vi "Temp Sweep Control.vi"() -> ()   [LabVIEW 2016, in "Transport.lvclass"]
uses:
  Transport.lvclass
  Control Experiment SM/Control Experiment SM.lvclass
  <userlib>/LevyLab/Levylab Instruments/Instrument Types/Cryostat/Instrument.Cryostat.lvclass
panel:
  out "Current State":string
  in  "Wait time":dbl
  in  "T Start (K)":i32=275
  in  "T Step (K)":i32=5
  in  "Number":i32=26
  out "sequence":string
  in  "simulate?":bool
  in  "Start":bool
  in  "OK":bool
  in  "Experiment Description":string
  in  "Experiment Folder (## - Description)":string="00 - test"
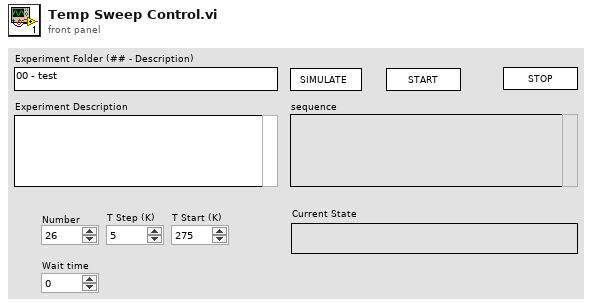
[diagram p1: front panel]
types:
  T1 = enum32{"Invalid", "Standard", "Closed", "Hidden", "Minimized", "Maximized"}
  T2 = enum32{"invalid app kind", "Development System", "Run Time System", "Student Edition", "Embedded LabVIEW", "Evaluation", "Custom"}
  T3 = cluster{"Core":cluster{"Current VI Reference":refnum<vi>, "Close Panel on Exit?":bool}, "C.E.":refnum<class "Control Experiment SM.lvclass">, "notifier":refnum<notifier>, "Lockin Start":timestamp, "Temp":dbl, "Wait time":dbl}
  T4 = cluster{"Current VI Reference":refnum<vi>, "Close Panel on Exit?":bool}
  T5 = typedef "Control Experiment SM.lvclass/Instruments--cluster.ctl" = cluster{"KH7008":refnum<class "Instrument.KH7008.lvclass">[], "Lockin":refnum<class "Instrument.Lockin.lvclass">, "Temperature":refnum<class "Instrument.Cryostat.lvclass">, "Magnet":refnum<class "Instrument.Cryostat.lvclass">, "Rotator":refnum<class "Instrument.Cryostat.lvclass">, "Level":refnum<class "Instrument.Cryostat.lvclass">, "Capacitance Bridge":refnum<class "Instrument.CBridge.lvclass">, "Optical Delay Line":refnum<class "Instrument.OpticalDelayLine.lvclass">, "Strain Cell":refnum<class "Instrument.Strain.lvclass">, "VNA":refnum<class "Instrument.VNA.lvclass">, "Voltage Source":refnum<class "Instrument.VSource.lvclass">}
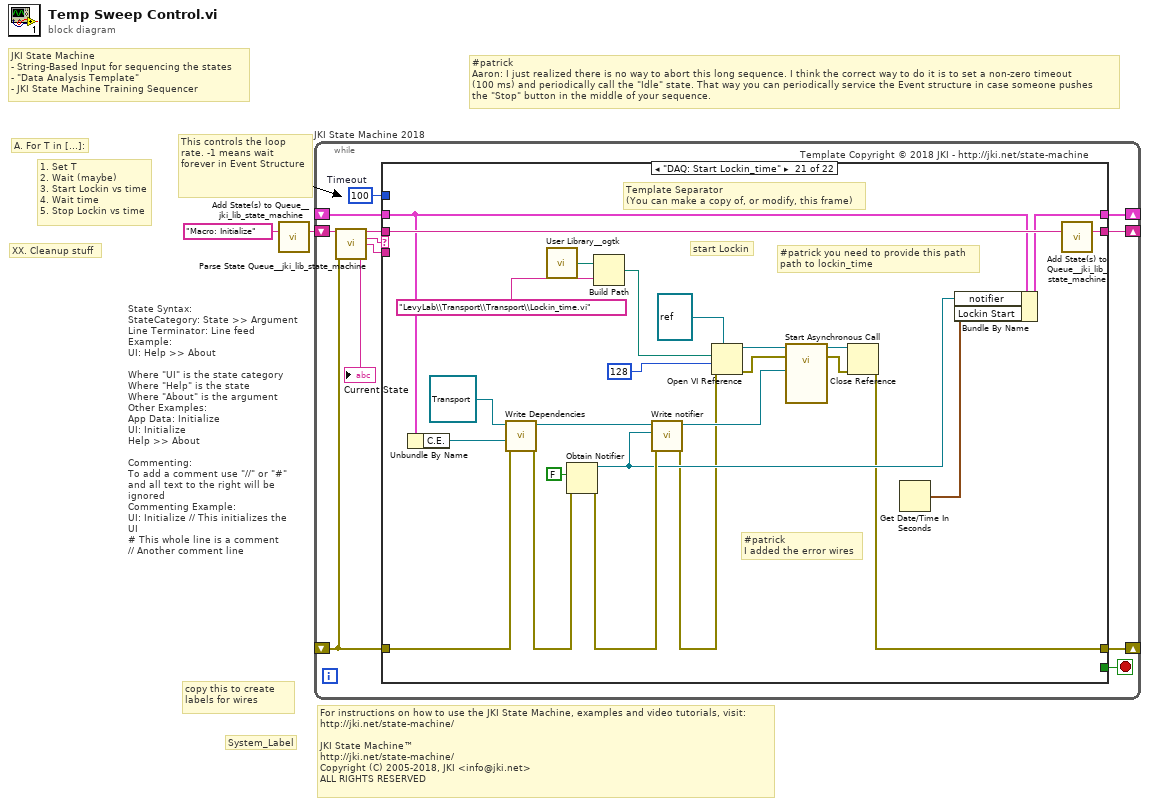
[diagram p0: block diagram]
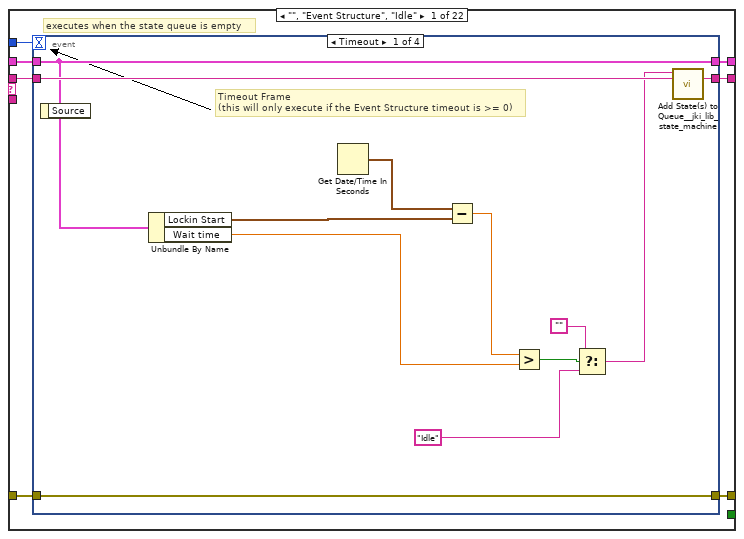
[diagram p2: hidden frame]
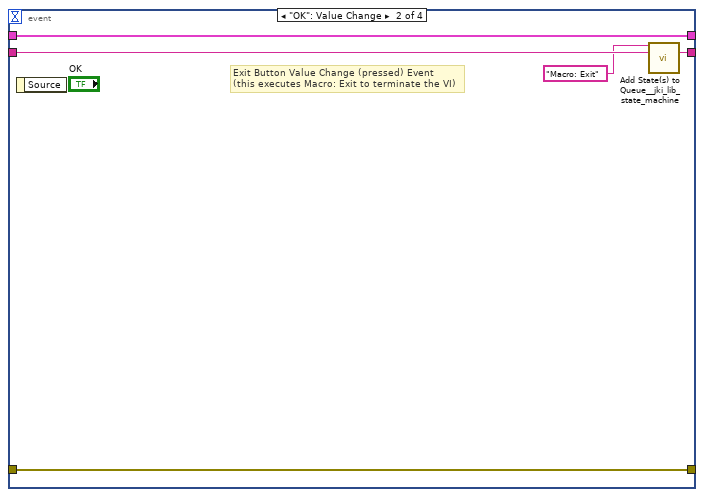
[diagram p3: hidden frame]
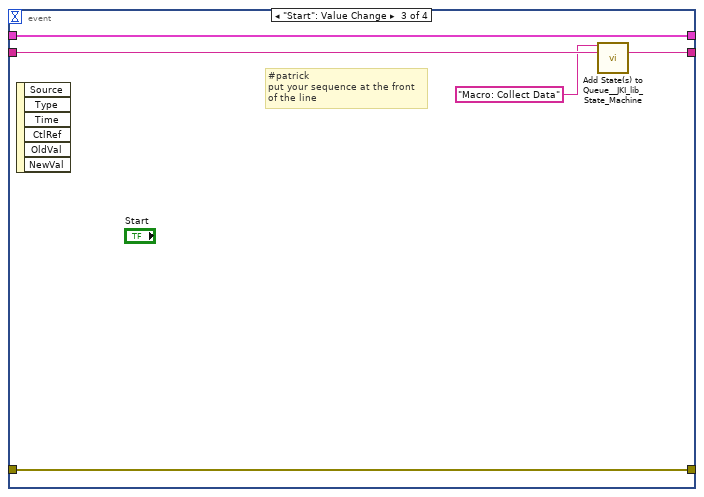
[diagram p4: hidden frame]
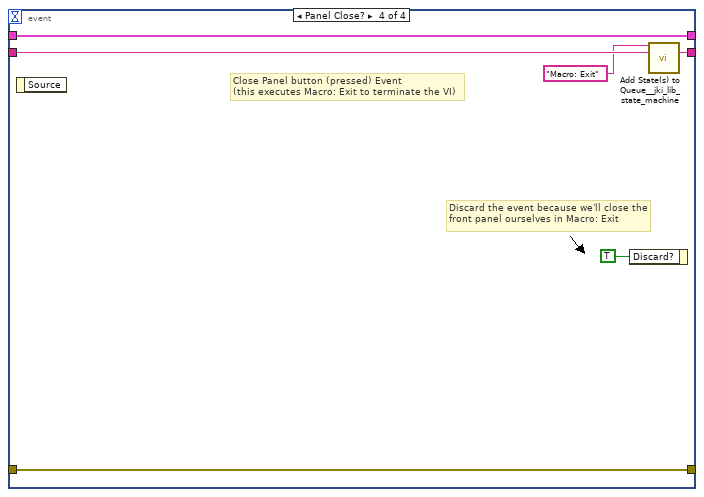
[diagram p5: hidden frame]
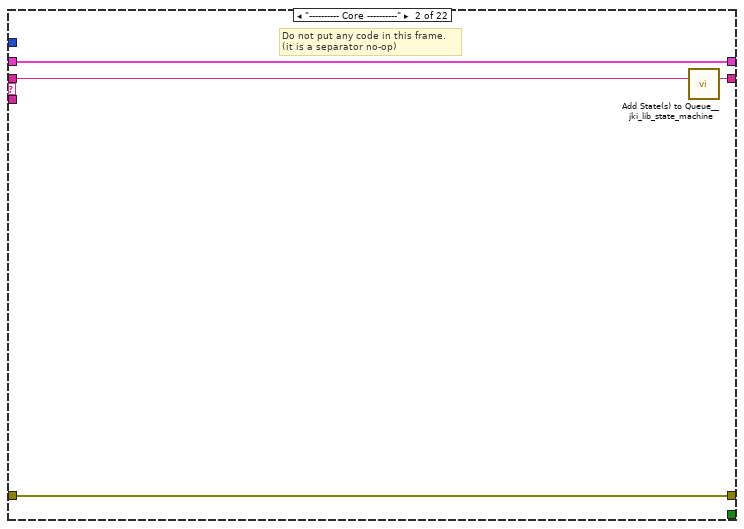
[diagram p6: hidden frame]
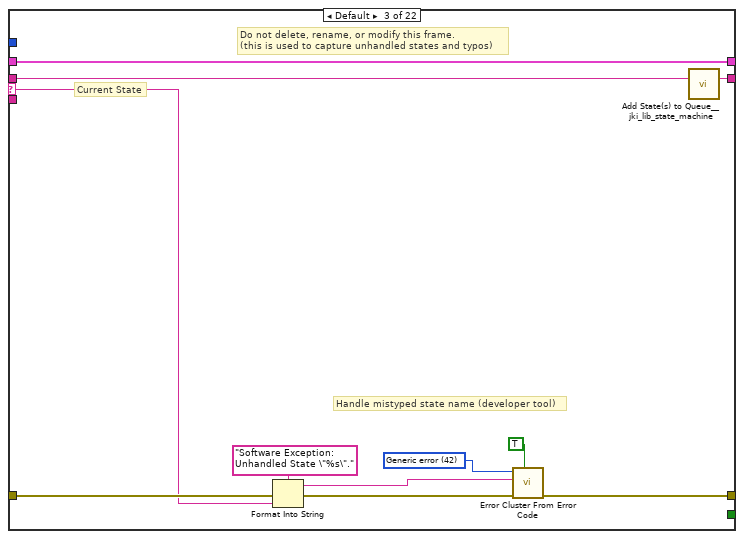
[diagram p7: hidden frame]
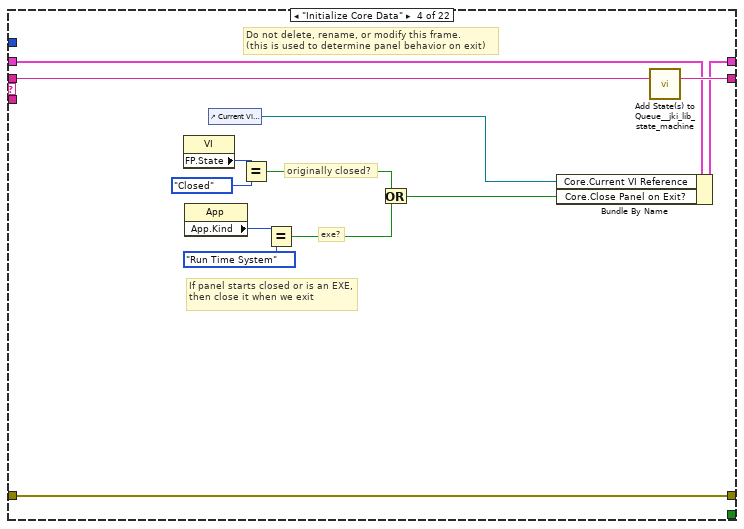
[diagram p8: hidden frame]
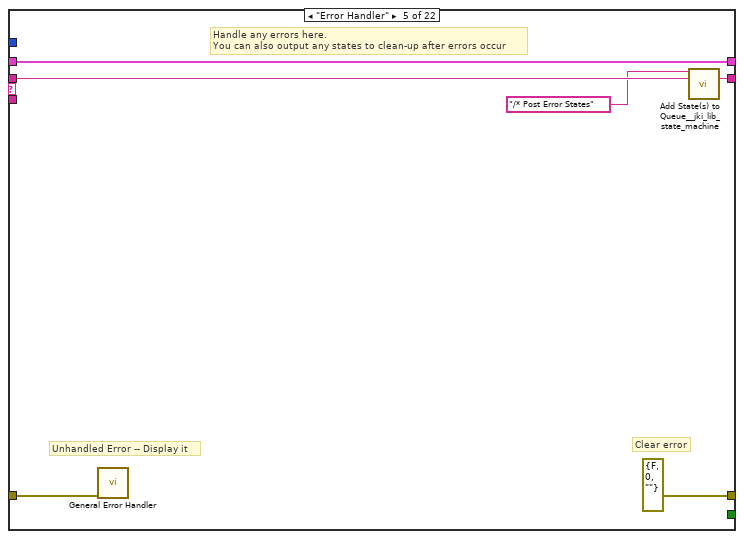
[diagram p9: hidden frame]
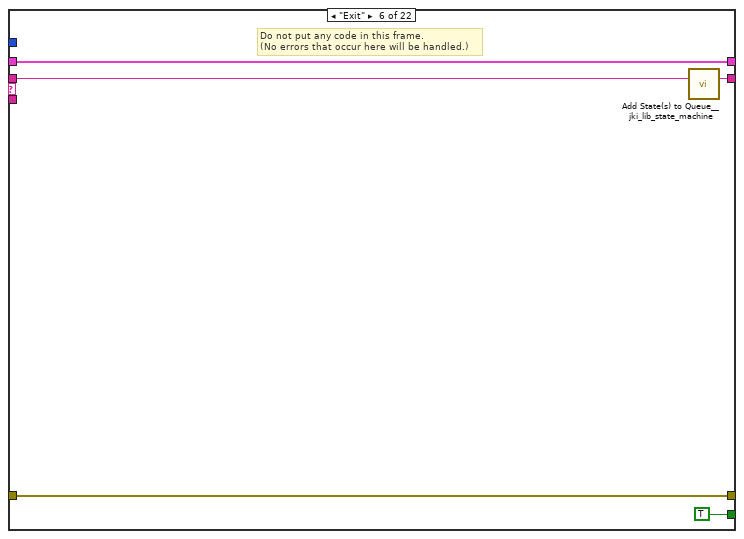
[diagram p10: hidden frame]
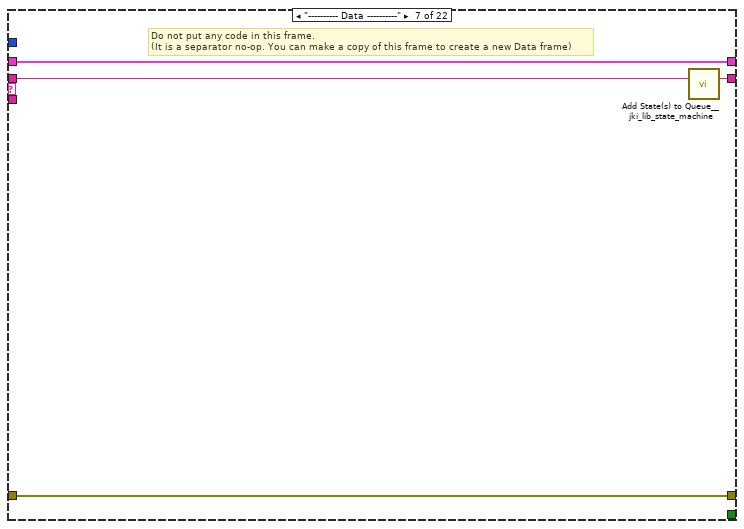
[diagram p11: hidden frame]
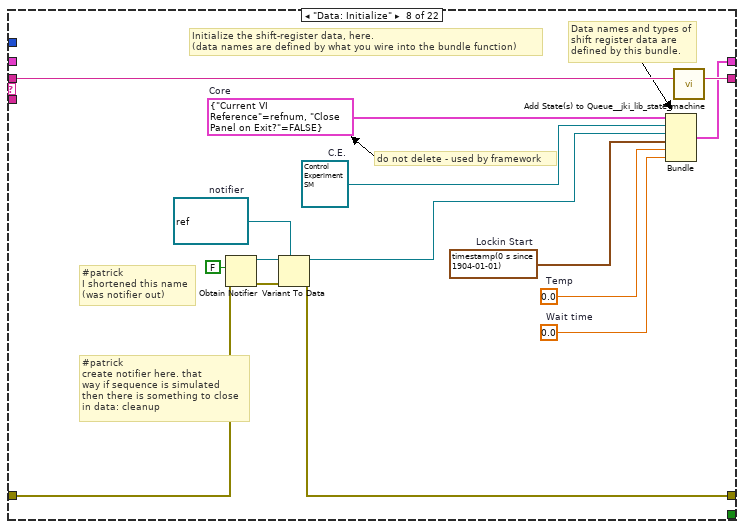
[diagram p12: hidden frame]
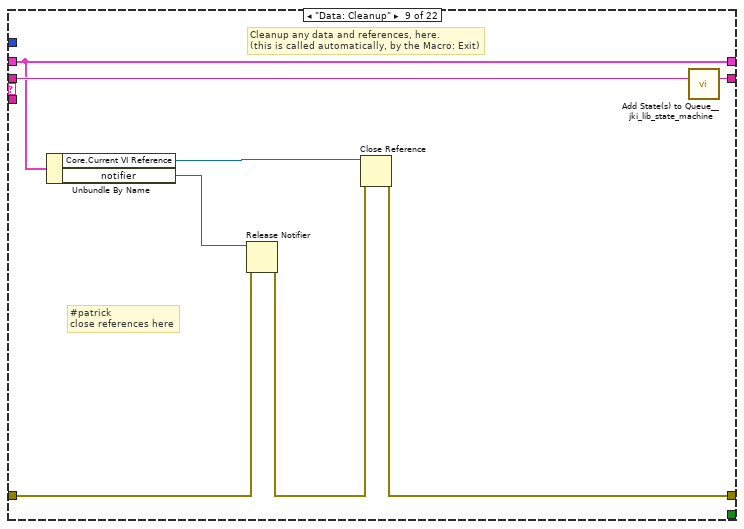
[diagram p13: hidden frame]
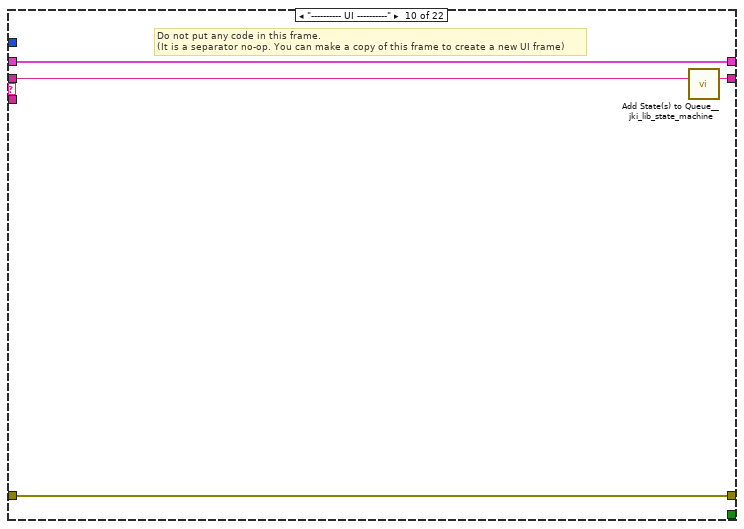
[diagram p14: hidden frame]
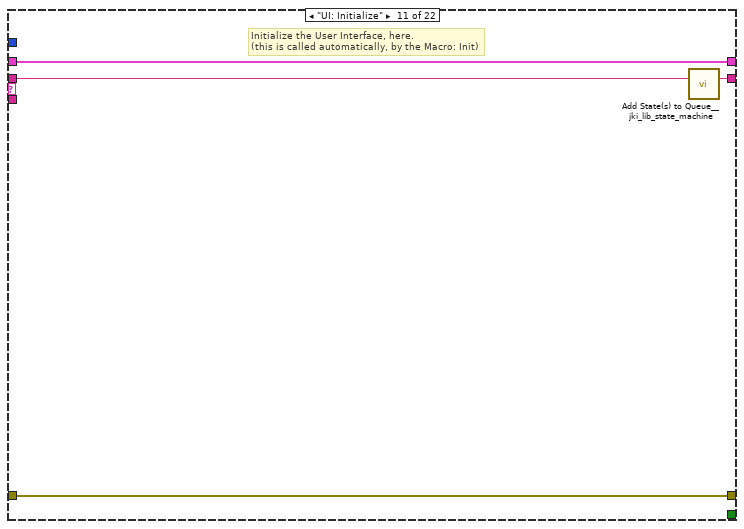
[diagram p15: hidden frame]
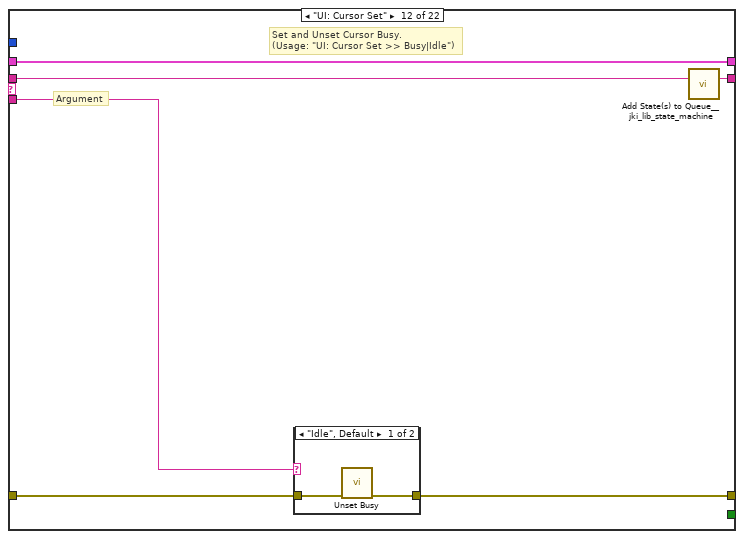
[diagram p16: hidden frame]
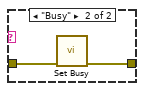
[diagram p17: hidden frame]
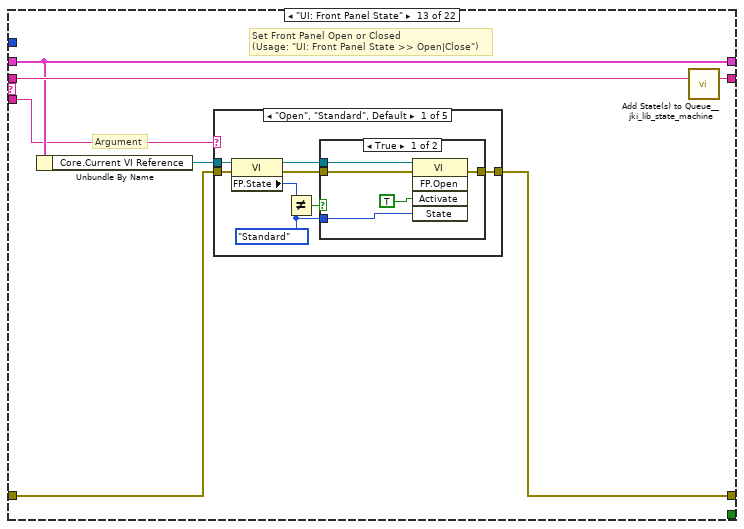
[diagram p18: hidden frame]
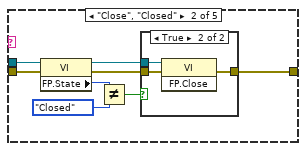
[diagram p20: hidden frame]
diagram:
  # "#patrick\nAaron: I just realized there is no way to abort this long sequence. I think the correct way to do it is to set a non-zero timeout\n(100 ms) and periodically call the \"Idle\" state. That way you can periodically service the Event structure in case someone pushes\nthe \"Stop\" button in the middle of your sequence."
  # "For instructions on how to use the JKI State Machine, examples and video tutorials, visit:\nhttp://jki.net/state-machine/\n\nJKI State Machine™\nhttp://jki.net/state-machine/\nCopyright (C) 2005-2018, JKI <info@jki.net>\nALL RIGHTS RESERVED"
  # "State Syntax:\nStateCategory: State >> Argument\nLine Terminator: Line feed\nExample:\nUI: Help >> About\n\nWhere \"UI\" is the state category\nWhere \"Help\" is the state\nWhere \"About\" is the argument\nOther Examples:\nApp Data: Initialize\nUI: Initialize\nHelp >> About\n\nCommenting:\nTo add a comment use \"//\" or \"#\" and all text to the right will be ignored\nCommenting Example:\nUI: Initialize // This initializes the UI\n# This whole line is a comment\n// Another comment line"
  # "copy this to create labels for wires"
  # "This controls the loop rate. -1 means wait forever in Event Structure"
  # "System_Label"
  # "JKI State Machine\n- String-Based Input for sequencing the states\n- \"Data Analysis Template\"\n- JKI State Machine Training Sequencer"
  # "XX. Cleanup stuff"
  # "A. For T in [...]:"
  # "1. Set T\n2. Wait (maybe)\n3. Start Lockin vs time\n4. Wait time\n5. Stop Lockin vs time"
  n1 = call <vilib>:"Add State(s) to Queue__jki_lib_state_machine.vi"("State(s) in (\"\")"="Macro: Initialize") -> ("States Out"=w2:string)  [unwired: 14 in]
  n2 = while "JKI State Machine 2018" {
    shift-right: [w6] -> _
    shift-left: _ -> [w5]
    shift-right: [w9] -> _
    shift-left: _ -> [w3]
    shift-right: [w8] -> _
    shift-left: w2 -> [w10]
    stop <- w7 stop-if-true
    w4 = 100  # Timeout
    # "Template Copyright © 2018 JKI - http://jki.net/state-machine"
    n3 = call <vilib>:"Parse State Queue__jki_lib_state_machine.vi"("State Queue"=w10, "Error In (no error)"=w3) -> ("Remaining States"=w12:string, "Current State"=w13:string, "Arguments"=w11:string)  [unwired: 11 in]
    "Current State" <- w13
    n4 = case shown="\"DAQ: Start Lockin_time\"" w13 {
      selector: w13 -> [_ _ w53 _ _ _ _ _ _ _ _ _ _ _ _ _ _ _ _ _ _ _]
      tunnel: w12 -> [w20 w52 w57 w76 w82 w87 w91 w106 w114 w118 w122 w128 w139 w208 w213 w226 w248 w252 w267 w284 w320 w327]
      tunnel: w11 -> [_ _ _ _ _ _ _ _ _ _ _ w123 w133 _ _ _ _ _ _ w279 _ _]
      tunnel: w5 -> [w18 w49 w55 w69 w79 w85 w88 _ w110 w115 w120 w126 w135 w205 w210 w223 w245 w249 w254 w278 w310 w325]
      tunnel: [w17 w50 w59 w73 errorcluster {"status"=FALSE, "code"=0, "source"=""} ("error out") w84 w89 w93 w111 w116 w119 w124 w136 w206 w211 w224 w246 w250 w258 w268 w300 w321] -> w9
      tunnel: w3 -> [w16 w50 w58 w73 w78 w84 w89 w94 w108 w116 w119 w125 w137 w206 w211 w224 w246 w250 w256 w276 w306 w322]
      tunnel: [w19 w51 w56 w75 w81 w86 w90 w105 w113 w117 w121 w127 w138 w207 w212 w225 w247 w251 w266 w283 w319 w326] -> w8
      tunnel: [_ _ _ _ _ TRUE _ _ _ _ _ _ _ _ _ _ _ _ _ _ _ _] -> w7
      tunnel: [w15 w49 w55 w74 w79 w85 w88 w104 w110 w115 w120 w126 w135 w205 w210 w223 w245 w249 w255 w277 w312 w325] -> w6
      tunnel: w4 -> [w14 _ _ _ _ _ _ _ _ _ _ _ _ _ _ _ _ _ _ _ _ _]
      frame "", "Event Structure", "Idle" {
        # "executes when the state queue is empty"
        n5 = event shown="[0] Timeout" {
          selector: _ -> [_ _ _ _]
          dyn-events: _ -> [_ _ _ _]
          timeout: w14 -> [_ _ _ _]
          tunnel: w20 -> [w32 w37 w40 w48]
          tunnel: [w31 w36 w39 w47] -> w19
          tunnel: w18 -> [w24 w34 w41 w45]
          tunnel: [w30 w35 w42 w46] -> w17
          tunnel: w16 -> [w30 w35 w42 w46]
          tunnel: [w24 w34 w41 w45] -> w15
          event Timeout {
            # "Timeout Frame\n(this will only execute if the Event Structure timeout is >= 0)"
            n6 = event-data() -> ()  [unwired: 1 in, 1 out]
            n7 = Unbundle By Name(w24) -> ("Lockin Start"=w22:timestamp, "Wait time"=w23:dbl)
            n8 = Get Date/Time In Seconds() -> (seconds since 1Jan1904=w29:timestamp)
            n9 = Subtract(x=w29, y=w22) -> (x-y=w28:dbl)
            n10 = Greater?(x=w28, y=w23) -> (0:w27:bool)
            n11 = Select(t="", s=w27, f="Idle") -> (s? t:f=w21:string)
            n12 = call <vilib>:"Add State(s) to Queue__jki_lib_state_machine.vi"("State(s) in Front (\"\")"=w21, "State(s) in (\"\")"=w32) -> ("States Out"=w31:string)  [unwired: 13 in]
          }
          event "OK": Value Change {
            # "Exit Button Value Change (pressed) Event\n(this executes Macro: Exit to terminate the VI)"
            n13 = event-data() -> ()  [unwired: 1 in, 1 out]
            n14 = call <vilib>:"Add State(s) to Queue__jki_lib_state_machine.vi"("State(s) in Front (\"\")"="Macro: Exit", "State(s) in (\"\")"=w37) -> ("States Out"=w36:string)  [unwired: 13 in]
          }
          event "Start": Value Change {
            # "#patrick\nput your sequence at the front\nof the line"
            n15 = event-data() -> ()  [unwired: 1 in, 6 out]
            n16 = call <vilib>:"Add State(s) to Queue__JKI_lib_State_Machine.vi"("State(s) in Front (\"\")"="Macro: Collect Data", "State(s) in (\"\")"=w40) -> ("States Out"=w39:string)  [unwired: 13 in]
          }
          event Panel Close? {
            # "Discard the event because we'll close the front panel ourselves in Macro: Exit"
            # "Close Panel button (pressed) Event\n(this executes Macro: Exit to terminate the VI)"
            n17 = event-data() -> ()  [unwired: 1 in, 1 out]
            n18 = event-data("Discard?"=TRUE) -> ()  [unwired: 1 in, 1 out]
            n19 = call <vilib>:"Add State(s) to Queue__jki_lib_state_machine.vi"("State(s) in Front (\"\")"="Macro: Exit", "State(s) in (\"\")"=w48) -> ("States Out"=w47:string)  [unwired: 13 in]
          }
        }
      }
      frame "---------- Core ----------" {
        # "Do not put any code in this frame.\n(it is a separator no-op)"
        n20 = call <vilib>:"Add State(s) to Queue__jki_lib_state_machine.vi"("State(s) in (\"\")"=w52) -> ("States Out"=w51:string)  [unwired: 14 in]
      }
      frame Default {
        w62 = 42 items=["No error", "Argument error", "Memory is full", "Out of zone", "End of file", "File already open", "Generic file I/O error", "File not found", "File permission error", "Disk is full", "Duplicate path", "Too many files open", "System feature not enabled", "Resource file not found", "Cannot add resource", "Resource not found", "Image not found", "Image memory error", "Pen does not exist", "Config type invalid", "Config token not found", "Config parse error", "Config memory error", "Bad external code format", "Bad external code offset", "External code not present", "Null window", "Destroy window error", "Null menu", "Print aborted", "Bad print record", "Print driver error", "Windows error during printing", "Memory error during printing", "Print dialog error", "Generic print error", "Invalid device refnum", "Device not found", "Device parameter error", "Device unit error", "Cannot open device", "Device call aborted", "Generic error", "Cancelled by user", "Object ID too low", "Object ID too high", "Object not in heap", "Unknown heap", "Unknown object (invalid DefProc)", "Unknown object (DefProc not in table)", "Message out of range", "Invalid (null) method", "Unknown message", "Manager call not supported", "Bad address", "Network operation in progress", "Network operation timed out", "Connection is busy", "Network attribute not supported", "Network error", "Address in use", "System out of memory", "Connection aborted", "Connection refused", "Not connected", "Already connected", "Connection closed", "Initialization error (interapplication manager)", "Bad occurrence", "Wait on unbound occurrence handler", "Occurrence queue overflow", "Datalog type conflict", "Unused", "Unrecognized type (interapplication manager)", "Memory corrupt", "Failed to make temporary DLL", "Old CIN version", "Drag socket not found", "Failed to load drop-object", "Failed to register OLE object", "Failed to release OLE object", "Format specifier type mismatch", "Unknown format specifier", "Too few format specifiers", "Too many format specifiers", "Scan failed", "Newer CIN version", "Error converting to variant", "Runtime menu error", "Password tampered", "Variant attribute not found", "Incompatible variant data type", "Event data is not available", "Event Store is not present", "Occurrence is not found", "Event Queue is not created", "Event info is not available", "Refnum passed is NULL", "Error retrieving Class GUID", "Error retrieving CoClass GUID", "Error retrieving TypeLib GUID.", "Bad built application magic bytes.", "Specific driver is different from the specific driver associated with the Logical Name.", "There is no session opened to the class driver.", "Max Error", "MAX - Error with config objects", "MAX - Error loading configuration", "MAX - Group not supported"]
        # "Current State"
        # "Do not delete, rename, or modify this frame.\n(this is used to capture unhandled states and typos)"
        # "Handle mistyped state name (developer tool)"
        n21 = Format Into String(format string="Software Exception: Unhandled State \"%s\"." ("message"), error in=w58, w53) -> (resulting string=w61:string, error out=w60:errorcluster)  [unwired: 1 in]
        n22 = call <vilib>:"Error Cluster From Error Code.vi"("show call chain? (False)"=TRUE, "error in (no error)"=w60, "error message (\"\")"=w61, "error code (0)"=w62) -> ("error out"=w59:errorcluster)  [unwired: 5 in]
        n23 = call <vilib>:"Add State(s) to Queue__jki_lib_state_machine.vi"("State(s) in (\"\")"=w57) -> ("States Out"=w56:string)  [unwired: 14 in]
      }
      frame "Initialize Core Data" {
        # "Do not delete, rename, or modify this frame.\n(this is used to determine panel behavior on exit)"
        # "originally closed?"
        # "exe?"
        # "If panel starts closed or is an EXE, then close it when we exit"
        n24 = property class="VI"() -> ("FP.State"=w66:T1)  [unwired: 2 in, 2 out]
        n25 = property class="App"() -> ("App.Kind"=w72:T2)  [unwired: 2 in, 2 out]
        n26 = control-ref of="Current VI Reference"() -> (w67:refnum<vi>)
        n27 = Equal?(x=w66, y=T1."Closed" ("Front Panel Window:State")) -> (x = y?=w64:bool)
        n28 = Equal?(x=w72, y=T2."Run Time System" ("Application:Kind")) -> (x = y?=w70:bool)
        n29 = Or(x=w64, y=w70) -> (x .or. y?=w68:bool)
        n30 = Bundle By Name(cluster=w69, "Core.Current VI Reference"=w67, "Core.Close Panel on Exit?"=w68) -> (w74:T3)
        n31 = call <vilib>:"Add State(s) to Queue__jki_lib_state_machine.vi"("State(s) in (\"\")"=w76) -> ("States Out"=w75:string)  [unwired: 14 in]
      }
      frame "Error Handler" {
        # "Unhandled Error -- Display it"
        # "Handle any errors here.\nYou can also output any states to clean-up after errors occur"
        # "Clear error"
        n32 = call <vilib>:"General Error Handler.vi"("error in (no error)"=w78) -> ()  [unwired: 10 in, 5 out]
        n33 = call <vilib>:"Add State(s) to Queue__jki_lib_state_machine.vi"("State(s) in Front (\"\")"="/* Post Error States", "State(s) in (\"\")"=w82) -> ("States Out"=w81:string)  [unwired: 13 in]
      }
      frame "Exit" {
        # "Do not put any code in this frame.\n(No errors that occur here will be handled.)"
        n34 = call <vilib>:"Add State(s) to Queue__jki_lib_state_machine.vi"("State(s) in (\"\")"=w87) -> ("States Out"=w86:string)  [unwired: 14 in]
      }
      frame "---------- Data ----------" {
        # "Do not put any code in this frame.\n(It is a separator no-op. You can make a copy of this frame to create a new Data frame)"
        n35 = call <vilib>:"Add State(s) to Queue__jki_lib_state_machine.vi"("State(s) in (\"\")"=w91) -> ("States Out"=w90:string)  [unwired: 14 in]
      }
      frame "Data: Initialize" {
        w92 = 0.0  # Wait time
        w100 = 0.0  # Temp
        w101 = timestamp(0 s since 1904-01-01)  # Lockin Start
        w96 = refnum<notifier> refnum  # notifier
        w102 = refnum<class "Control Experiment SM.lvclass"> refnum  # C.E.
        w103 = T4 {"Current VI Reference"=refnum, "Close Panel on Exit?"=FALSE}  # Core
        # "#patrick\ncreate notifier here. that\nway if sequence is simulated\nthen there is something to close\nin data: cleanup"
        # "#patrick\nI shortened this name\n(was notifier out)"
        # "do not delete - used by framework"
        # "Data names and types of shift register data are defined by this bundle."
        # "Initialize the shift-register data, here.\n(data names are defined by what you wire into the bundle function)"
        n36 = Obtain Notifier(notification data type=FALSE, error in (no error)=w94) -> (notifier out=w97:refnum<notifier>, error out=w98:errorcluster)  [unwired: 2 in, 1 out]
        n37 = Variant To Data(error in=w98, type=w96, Variant=w97) -> (data=w95:refnum<notifier>, error out=w93:errorcluster)
        n38 = Bundle("Core"=w103, "C.E."=w102, "notifier"=w95, "Lockin Start"=w101, "Temp"=w100, "Wait time"=w92) -> (w104:T3)  [unwired: 1 in]
        n39 = call <vilib>:"Add State(s) to Queue__jki_lib_state_machine.vi"("State(s) in (\"\")"=w106) -> ("States Out"=w105:string)  [unwired: 14 in]
      }
      frame "Data: Cleanup" {
        # "#patrick\nclose references here"
        # "Cleanup any data and references, here.\n(this is called automatically, by the Macro: Exit)"
        n40 = Unbundle By Name(w110) -> ("Core.Current VI Reference"=w112:refnum<vi>, "notifier"=w109:refnum<notifier>)
        n41 = Release Notifier(notifier=w109, error in (no error)=w108) -> (error out=w107:errorcluster)  [unwired: 1 in, 2 out]
        n42 = Close Reference(reference=w112, error in (no error)=w107) -> (error out=w111:errorcluster)
        n43 = call <vilib>:"Add State(s) to Queue__jki_lib_state_machine.vi"("State(s) in (\"\")"=w114) -> ("States Out"=w113:string)  [unwired: 14 in]
      }
      frame "---------- UI ----------" {
        # "Do not put any code in this frame.\n(It is a separator no-op. You can make a copy of this frame to create a new UI frame)"
        n44 = call <vilib>:"Add State(s) to Queue__jki_lib_state_machine.vi"("State(s) in (\"\")"=w118) -> ("States Out"=w117:string)  [unwired: 14 in]
      }
      frame "UI: Initialize" {
        # "Initialize the User Interface, here.\n(this is called automatically, by the Macro: Init)"
        n45 = call <vilib>:"Add State(s) to Queue__jki_lib_state_machine.vi"("State(s) in (\"\")"=w122) -> ("States Out"=w121:string)  [unwired: 14 in]
      }
      frame "UI: Cursor Set" {
        # "Argument"
        # "Set and Unset Cursor Busy.\n(Usage: \"UI: Cursor Set >> Busy|Idle\")"
        n46 = case shown="\"Idle\", Default" w123 {
          tunnel: w125 -> [w130 w132]
          tunnel: [w129 w131] -> w124
          frame "Idle", Default {
            n47 = call <vilib>:"Unset Busy.vi"("error in (no error)"=w130) -> ("error out"=w129:errorcluster)  [unwired: 10 in]
          }
          frame "Busy" {
            n48 = call <vilib>:"Set Busy.vi"("error in (no error)"=w132) -> ("error out"=w131:errorcluster)  [unwired: 9 in, 1 out]
          }
        }
        n49 = call <vilib>:"Add State(s) to Queue__jki_lib_state_machine.vi"("State(s) in (\"\")"=w128) -> ("States Out"=w127:string)  [unwired: 14 in]
      }
      frame "UI: Front Panel State" {
        # "Argument"
        # "Set Front Panel Open or Closed\n(Usage: \"UI: Front Panel State >> Open|Close\")"
        n50 = Unbundle By Name(w135) -> ("Core.Current VI Reference"=w134:refnum<vi>)
        n51 = case shown="\"Open\", \"Standard\", Default" w133 {
          tunnel: w137 -> [w145 w160 w171 w184 w197]
          tunnel: [w147 w161 w173 w186 w199] -> w136
          tunnel: w134 -> [w146 w158 w172 w185 w198]
          frame "Open", "Standard", Default {
            w140 = T1."Standard" ("State")
            n52 = property class="VI"(reference=w146, error in=w145) -> (reference out=w143:refnum<vi>, error out=w144:errorcluster, "FP.State"=w142:T1)
            n53 = Not Equal?(x=w142, y=w140) -> (x != y?=w141:bool)
            n54 = case shown="True" w141 {
              tunnel: [w151 w153] -> w147
              tunnel: w144 -> [w150 w153]
              tunnel: w143 -> [w149 _]
              tunnel: w140 -> [w148 _]
              frame True {
                n55 = invoke class="VI" method="FP.Open"(reference=w149, error in=w150, "Activate"=TRUE, "State"=w148) -> (error out=w151:errorcluster)  [unwired: 1 in, 4 out]
              }
              frame False {
              }
            }
          }
          frame "Close", "Closed" {
            n56 = property class="VI"(reference=w158, error in=w160) -> (reference out=w157:refnum<vi>, error out=w159:errorcluster, "FP.State"=w155:T1)
            n57 = Not Equal?(x=w155, y=T1."Closed" ("Front Panel Window:State")) -> (x != y?=w154:bool)
            n58 = case shown="True" w154 {
              tunnel: [w162 w165] -> w161
              tunnel: w159 -> [w162 w164]
              tunnel: w157 -> [_ w163]
              frame False {
              }
              frame True {
                n59 = invoke class="VI" method="FP.Close"(reference=w163, error in=w164) -> (error out=w165:errorcluster)  [unwired: 1 in, 2 out]
              }
            }
          }
          frame "Hidden", "Hide" {
            w166 = T1."Hidden" ("State")
            n60 = property class="VI"(reference=w172, error in=w171) -> (reference out=w169:refnum<vi>, error out=w170:errorcluster, "FP.State"=w168:T1)
            n61 = Not Equal?(x=w168, y=w166) -> (x != y?=w167:bool)
            n62 = case shown="True" w167 {
              tunnel: [w177 w178] -> w173
              tunnel: w170 -> [w176 w178]
              tunnel: w169 -> [w175 _]
              tunnel: w166 -> [w174 _]
              frame True {
                n63 = invoke class="VI" method="FP.Open"(reference=w175, error in=w176, "State"=w174) -> (error out=w177:errorcluster)  [unwired: 2 in, 4 out]
              }
              frame False {
              }
            }
          }
          frame "Minimize", "Minimized" {
            w179 = T1."Minimized" ("State")
            n64 = property class="VI"(reference=w185, error in=w184) -> (reference out=w182:refnum<vi>, error out=w183:errorcluster, "FP.State"=w181:T1)
            n65 = Not Equal?(x=w181, y=w179) -> (x != y?=w180:bool)
            n66 = case shown="True" w180 {
              tunnel: [w190 w191] -> w186
              tunnel: w183 -> [w189 w191]
              tunnel: w182 -> [w188 _]
              tunnel: w179 -> [w187 _]
              frame True {
                n67 = invoke class="VI" method="FP.Open"(reference=w188, error in=w189, "State"=w187) -> (error out=w190:errorcluster)  [unwired: 2 in, 4 out]
              }
              frame False {
              }
            }
          }
          frame "Maximize", "Maximized" {
            w192 = T1."Maximized" ("State")
            n68 = property class="VI"(reference=w198, error in=w197) -> (reference out=w195:refnum<vi>, error out=w196:errorcluster, "FP.State"=w194:T1)
            n69 = Not Equal?(x=w194, y=w192) -> (x != y?=w193:bool)
            n70 = case shown="True" w193 {
              tunnel: [w203 w204] -> w199
              tunnel: w196 -> [w202 w204]
              tunnel: w195 -> [w201 _]
              tunnel: w192 -> [w200 _]
              frame True {
                n71 = invoke class="VI" method="FP.Open"(reference=w201, error in=w202, "State"=w200) -> (error out=w203:errorcluster)  [unwired: 2 in, 4 out]
              }
              frame False {
              }
            }
          }
        }
        n72 = call <vilib>:"Add State(s) to Queue__jki_lib_state_machine.vi"("State(s) in (\"\")"=w139) -> ("States Out"=w138:string)  [unwired: 14 in]
      }
      frame "---------- Macro ----------" {
        # "Do not put any code in this frame.\n(It is a separator no-op. You can make a copy of this frame to create a new Macro frame)"
        n73 = call <vilib>:"Add State(s) to Queue__jki_lib_state_machine.vi"("State(s) in (\"\")"=w208) -> ("States Out"=w207:string)  [unwired: 14 in]
      }
      frame "Macro: Initialize" {
        w209 = "Data: Initialize\nInitialize Core Data\nUI: Initialize\nUI: Front Panel State >> Open"  # Data: Initialize Initialize Core Data UI: Initialize UI: Front Panel State >> Open
        # "Initialization Macro\n(This is called once, when the VI starts)"
        n74 = call <vilib>:"Add State(s) to Queue__jki_lib_state_machine.vi"("State(s) in Front (\"\")"=w209, "State(s) in (\"\")"=w213) -> ("States Out"=w212:string)  [unwired: 13 in]
      }
      frame "Macro: Collect Data" {
        # "#patrick\nyou might want this program\nto terminate when finished?"
        # "#patrick\nyou need a way to verify\nwhat sequences will run. This is\nsimplest way to see.\nBy running this I don't see a\nstate called \"Check Temp\""
        # "#patrick\nput your sequence at the front"
        # "#patrick\nThis is good. I like the loop to create your state sequence. I would probably add pauses so you can service the event queue\n(ie, how would you pause or terminate this seqeunce?)\nIn the future Temperature Start, Step, N, can be controls. Or set from the front panel via string"
        # "#patrick you probably\nwant to initalize this register"
        # "Do not put any code in this frame.\n(It is a separator no-op. You can make a copy of this frame to create a new Macro frame)"
        n75 = for {
          N: "Number" -> [_]
          shift-right: [w227] -> w216
          shift-left: "" ("States Out") -> [w231]
          i -> [w236]
          n76 = Multiply(x="T Step (K)", y=w236) -> (x*y=w237:i32)
          n77 = Add(x="T Start (K)", y=w237) -> (x+y=w234:i32)
          n78 = Format Into String(format string=" %d", initial string="DAQ: Set Temp >>", w234) -> (resulting string=w229:string)  [unwired: 1 in, 1 out]
          n79 = call <vilib>:"Add State(s) to Queue__jki_lib_state_machine.vi"("State(s) in Front (\"\")"=w229, "State(s) at Back (\"\")"="DAQ: Start Lockin_time\nIdle\nDAQ: Stop Lockin_time") -> ("States Out"=w230:string)  [unwired: 13 in]
          n80 = call <vilib>:"Add State(s) to Queue__jki_lib_state_machine.vi"("State(s) in (\"\")"=w231, "State(s) at Back (\"\")"=w230) -> ("States Out"=w227:string)  [unwired: 13 in]
        }
        n81 = call <vilib>:"Add State(s) to Queue__jki_lib_state_machine.vi"("State(s) in Front (\"\")"="DAQ: Init", "State(s) in (\"\")"=w216, "State(s) at Back (\"\")"="//Macro: Exit") -> ("States Out"=w217:string)  [unwired: 12 in]
        "sequence" <- w217
        n82 = Select(t="", s="simulate?", f=w217) -> (s? t:f=w220:string)
        n83 = call <vilib>:"Add State(s) to Queue__jki_lib_state_machine.vi"("State(s) in Front (\"\")"=w220, "State(s) in (\"\")"=w226) -> ("States Out"=w225:string)  [unwired: 13 in]
      }
      frame "Macro: Exit" {
        # "Exit Macro\n(This is called once, when the VI exits)"
        n84 = Unbundle By Name(w245) -> ("Core.Close Panel on Exit?"=w244:bool)
        n85 = Select(t="UI: Front Panel State >> Close", s=w244, f="") -> (s? t:f=w241:string)
        n86 = call <vilib>:"Add State(s) to Queue__jki_lib_state_machine.vi"("State(s) in (\"\")"=w241, "State(s) at Back (\"\")"="Data: Cleanup\nDAQ: Stop Lockin\nExit") -> ("States Out"=w239:string)  [unwired: 13 in]
        n87 = call <vilib>:"Add State(s) to Queue__jki_lib_state_machine.vi"("State(s) in Front (\"\")"=w239, "State(s) in (\"\")"=w248) -> ("States Out"=w247:string)  [unwired: 13 in]
      }
      frame "---------- DAQ ----------" {
        # "Template Separator\n(You can make a copy of, or modify, this frame)"
        n88 = call <vilib>:"Add State(s) to Queue__jki_lib_state_machine.vi"("State(s) in (\"\")"=w252) -> ("States Out"=w251:string)  [unwired: 14 in]
      }
      frame "DAQ: Init" {
        # "AA. Startup stuff"
        # "Your code here.\n(You can make a copy of, or modify, this frame)"
        n89 = call "Control Experiment FGV.vi"("Function"=enum16{"read", "write"}."read", "error in (no error)"=w256) -> ("error out"=w259:errorcluster, "Control Experiment.lvclass out"=w263:refnum<class "Control Experiment SM.lvclass">)  [unwired: 8 in]
        n90 = call "Write Experiment Description.vi"("error in (no error)"=w259, "Experiment Description"="Experiment Description", "Control Experiment in"=w263) -> ("error out"=w257:errorcluster, "Control Experiment out"=w265:refnum<class "Control Experiment SM.lvclass">)  [unwired: 7 in]
        n91 = call "Write Experiment Folder.vi"("error in (no error)"=w257, "Experiment Folder"="Experiment Folder (## - Description)", "Control Experiment in"=w265) -> ("error out"=w258:errorcluster, "Control Experiment out"=w260:refnum<class "Control Experiment SM.lvclass">)  [unwired: 7 in]
        n92 = Bundle By Name(cluster=w254, "C.E."=w260, "Wait time"="Wait time") -> (w255:T3)
        n93 = call <vilib>:"Add State(s) to Queue__jki_lib_state_machine.vi"("State(s) in (\"\")"=w267) -> ("States Out"=w266:string)  [unwired: 14 in]
      }
      frame "DAQ: Set Temp" {
        # "#patrick\nfuture upgrade can be to put the Temperature class onto the data cluster\nread it from C.E. in data initialize, for example."
        # "Your code here.\n(You can make a copy of, or modify, this frame)"
        n94 = Unbundle By Name(w278) -> ("C.E."=w282:refnum<class "Control Experiment SM.lvclass">)
        n95 = call "Read Instruments.vi"("error in (no error)"=w276, "Control Experiment in"=w282) -> ("error out"=w275:errorcluster, "Instruments"=w281:T5, "Control Experiment out"=w273:refnum<class "Control Experiment SM.lvclass">)  [unwired: 7 in]
        n96 = Unbundle By Name(w281) -> ("Temperature"=w280:refnum<class "Instrument.Cryostat.lvclass">)
        n97 = Scan From String(input string=w279) -> (output 1=w271:dbl)  [unwired: 4 in, 3 out]
        n98 = call-dynamic "Set Temperature.vi"("error in (no error)"=w275, "Rate (K/min)"=2.0, "Temperature (K)"=w271, "Instrument.Cryostat in"=w280) -> ("error out"=w269:errorcluster, "Instrument.Cryostat out"=w272:refnum<class "Instrument.Cryostat.lvclass">)  [unwired: 6 in]
        n99 = while {
          tunnel: w272 -> [w289]
          tunnel: w271 -> [w288]
          tunnel: [w288] -> w270
          tunnel: w269 -> [w287]
          tunnel: [w285] -> w268
          stop <- w291 stop-if-true
          n100 = call <userlib>:"Wait (ms)__ogtk.vi"("error in (no error)"=w287, "milliseconds to wait"=u32 1000) -> ("error out"=w286:errorcluster)  [unwired: 8 in, 1 out]
          n101 = call-dynamic "Get Temperature.vi"("error in (no error)"=w286, "Instrument.Cryostat in"=w289) -> ("error out"=w285:errorcluster, "Temperature (K)"=w290:dbl)  [unwired: 5 in, 3 out]
          n102 = Subtract(x=w290, y=w288) -> (x-y=w295:dbl)
          n103 = Absolute Value(x=w295) -> (abs(x)=w294:dbl)
          n104 = Less Or Equal?(x=w294, y=0.01) -> (x <= y?=w291:bool)
        }
        n105 = Bundle By Name(cluster=w278, "C.E."=w273, "Temp"=w270) -> (w277:T3)
        n106 = call <vilib>:"Add State(s) to Queue__jki_lib_state_machine.vi"("State(s) in (\"\")"=w284) -> ("States Out"=w283:string)  [unwired: 14 in]
      }
      frame "DAQ: Start Lockin_time" {
        # "#patrick\nI added the error wires"
        # "start Lockin"
        # "#patrick you need to provide this path\npath to lockin_time"
        # "Template Separator\n(You can make a copy of, or modify, this frame)"
        n107 = Unbundle By Name(w310) -> ("C.E."=w309:refnum<class "Control Experiment SM.lvclass">)
        n108 = call "Write Dependencies.vi"("error in (no error)"=w306, "Control Experiment"=w309, "Transport in"=refnum<class "Transport.lvclass"> refnum) -> ("error out"=w305:errorcluster, "Transport out"=w311:refnum<class "Transport.lvclass">)  [unwired: 7 in]
        n109 = call <userlib>:"User Library__ogtk.vi"() -> ("User Library (+ Relative)"=w299:path)  [unwired: 1 in]
        n110 = Obtain Notifier(notification data type=FALSE, error in (no error)=w305) -> (notifier out=w304:refnum<notifier>, error out=w307:errorcluster)  [unwired: 2 in, 1 out]
        n111 = Build Path(base path=w299, name or relative path="LevyLab\\Transport\\Transport\\Lockin_time.vi") -> (appended path=w298:path)
        n112 = call "Write notifier.vi"("error in (no error)"=w307, "notifier"=w304, "Transport in"=w311) -> ("error out"=w301:errorcluster, "Transport out"=w314:refnum<class "Transport.lvclass">)  [unwired: 7 in]
        n113 = Open VI Reference(type specifier VI Refnum (for type only)=refnum<vi> refnum, vi path=w298, options=128, error in (no error)=w301) -> (vi reference=w317:refnum<vi>, error out=w302:errorcluster)  [unwired: 2 in]
        n114 = call-by-ref "Start Asynchronous Call"(reference=w317, error in=w302, "Transport"=w314) -> (reference out=w315:refnum<vi>, error out=w303:errorcluster)  [unwired: 9 in, 2 out]
        n115 = Close Reference(reference=w315, error in (no error)=w303) -> (error out=w300:errorcluster)
        n116 = Get Date/Time In Seconds() -> (seconds since 1Jan1904=w308:timestamp)
        n117 = Bundle By Name(cluster=w310, "notifier"=w304, "Lockin Start"=w308) -> (w312:T3)
        n118 = call <vilib>:"Add State(s) to Queue__jki_lib_state_machine.vi"("State(s) in (\"\")"=w320) -> ("States Out"=w319:string)  [unwired: 14 in]
      }
      frame "DAQ: Stop Lockin_time" {
        # "#patrick\nwire error terminals"
        # "stop lockin"
        # "Template Separator\n(You can make a copy of, or modify, this frame)"
        n119 = Unbundle By Name(w325) -> ("notifier"=w324:refnum<notifier>)
        n120 = Send Notification(notification=TRUE, notifier=w324, error in (no error)=w322) -> (error out=w321:errorcluster)  [unwired: 1 out]
        n121 = call <vilib>:"Add State(s) to Queue__jki_lib_state_machine.vi"("State(s) in (\"\")"=w327) -> ("States Out"=w326:string)  [unwired: 14 in]
      }
    }
  }
